vi "FIFO.vi"() -> ()   [LabVIEW 2019]
uses:
  <vilib>/rvi/Emulation/niFpgaGetClockAttributes.vi
  <vilib>/rvi/Emulation/niFpgaSctlEmulationGetInTimedLoop.vi
  <vilib>/rvi/Emulation/niFpgaEmulationReportErrorSimple.vi
  <vilib>/rvi/eio/common/nirviEmuTemplateMethod_errors.vi
  <vilib>/rvi/DataTransferAndStorage/Container/Common/niFpgaContainerExecOnDevCompGetState.vi
  <vilib>/rvi/Emulation/niFpgaEmulationIsFPGAContextNoSignature.vi
  <vilib>/rvi/errors/niFpgaSetErrorForExecOnDevCompSimple.vi
  <vilib>/rvi/eio/common/nirviEmuReportErrorAndStop.vi
  <vilib>/rvi/DataTransferAndStorage/Container/Common/niFpgaContainerGetUniqueNameForEmu.vi
  <vilib>/rvi/FIFO/Fifo_Resource/nirvififoEmulationSetSize.vi
  <vilib>/rvi/FIFO/Fifo_Resource/nirviFifoEmulationQueueMgr.vi
  <instcachedir>/0/nirviFifoEmulationQueueMgr_E5CAEC123FF24DC58D834DCA3CDAA9B5.lvgen/nirviFifoEmulationQueueMgr_E5CAEC123FF24DC58D834DCA3CDAA9B5_002.vi
  <vilib>/rvi/FIFO/Fifo_Resource/nirvififoEmulationDetermineInputValidOut.vi
  <vilib>/rvi/FIFO/Fifo_Resource/nirvififoEmulationCreateLock.vi
  <vilib>/rvi/Emulation/niFpgaProcessEmulError.vi
  <vilib>/rvi/FIFO/Fifo_Resource/nirvififoEmulationObtainLock.vi
  <vilib>/rvi/FIFO/Fifo_Resource/nirvififoEmulationReleaseLock.vi
  <vilib>/rvi/occurrence/nirviWaitOnOccurrenceBase.vi
  <vilib>/rvi/errors/nirviReportUnexpectedCaseInternalError.vi
  <vilib>/rvi/errors/nirviReportUnexpectedCaseInternalError (U32).vi
  <vilib>/Utility/error.llb/Clear Errors.vi
  <vilib>/rvi/interface/RandomDataEmulation/niFpgaRandomDataHandleErrors.vi
  <instcachedir>/0/nirviFifoEmulationQueueMgr_E5CAEC123FF24DC58D834DCA3CDAA9B5.lvgen/nirviFifoEmulationQueueMgr_E5CAEC123FF24DC58D834DCA3CDAA9B5_000.vi
  <instcachedir>/0/nirviFifoEmulationQueueMgr_E5CAEC123FF24DC58D834DCA3CDAA9B5.lvgen/nirviFifoEmulationQueueMgr_E5CAEC123FF24DC58D834DCA3CDAA9B5_001.vi
  <vilib>/rvi/Emulation/niFpgaCriticalErrorInLSC.vi
  <vilib>/eio/EIONode/EIONode.xnode
  <vilib>/rvi/DataTransferAndStorage/Container/XNode/niFpgaContainer.xnode
  <vilib>/rvi/FIFO/Fifo_Resource/niFpgaFifoEmulationRefIn.vi
panel:
  out "Laser":i16
  in  "stop":bool
  out "volt":i16
  out "Count":u32 caption="Tick Count(uSec)"
  out "Load":u16
  in  "Count(uSec)":u32
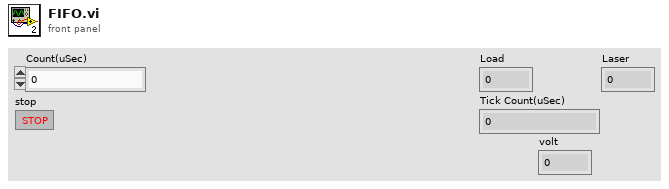
[diagram p1: front panel]
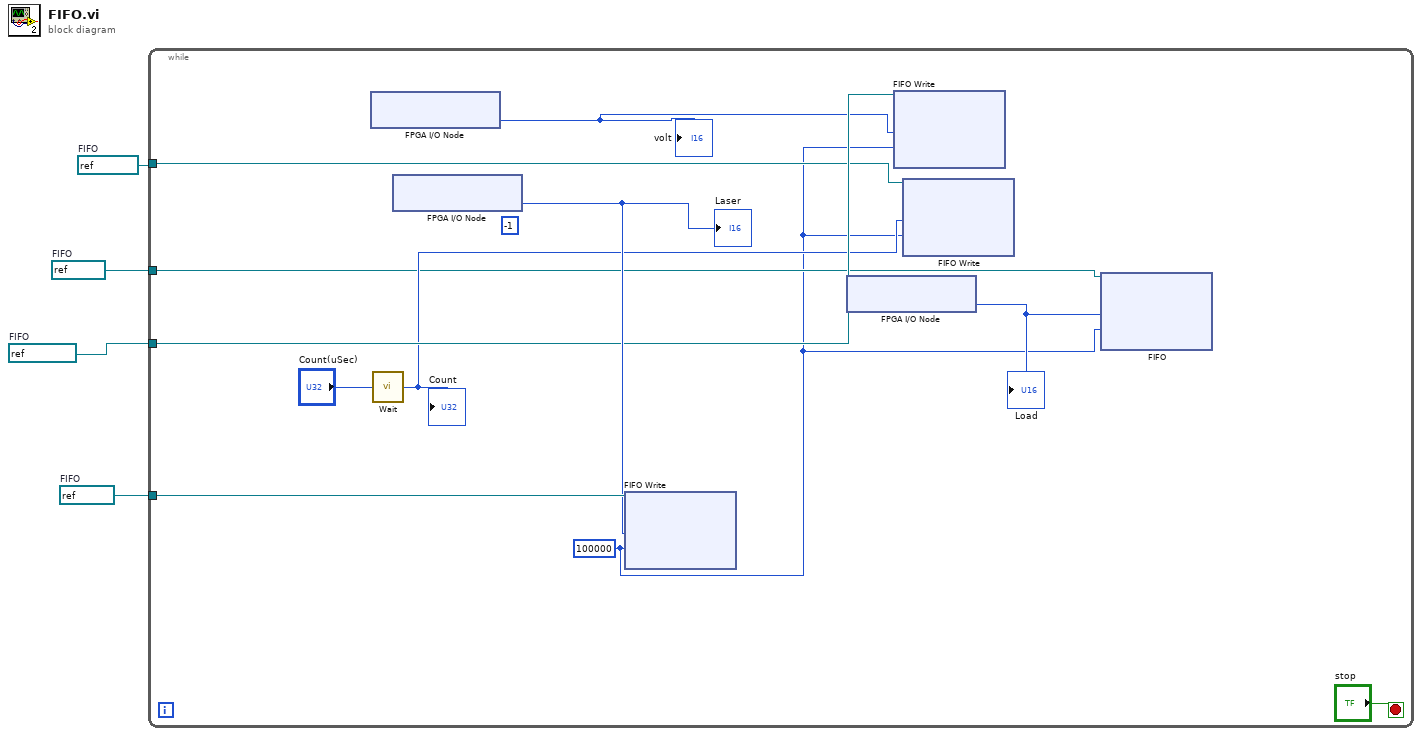
[diagram p0: block diagram]
diagram:
  w1 = refnum<k21> "Load"  # FIFO
  w2 = refnum<k21> "Count"  # FIFO
  w3 = refnum<k21> "Voltage"  # FIFO
  w4 = refnum<k21> "Laser"  # FIFO
  n1 = while {
    tunnel: w4 -> [w13]
    tunnel: w3 -> [w11]
    tunnel: w2 -> [w9]
    tunnel: w1 -> [w7]
    stop <- "stop" stop-if-true
    w5 = 100000 ("Timeout")
    (unwired) -1
    n2 = xnode "FPGA I/O Node"() -> ("ConnectorC/AI0"=w10:i16)  [unwired: 1 in, 1 out]
    "volt" <- w10
    n3 = call "Wait"("Count(uSec)"="Count(uSec)") -> ("Tick Count(uSec)"=w8:u32)
    "Count" <- w8
    n4 = xnode "FPGA I/O Node"() -> ("ConnectorC/AI1"=w12:i16)  [unwired: 1 in, 1 out]
    "Laser" <- w12
    n5 = xnode ("FIFO Write")("Element"=w12, "Timeout"=w5, "FIFO In"=w13) -> ()  [unwired: 2 out]
    n6 = xnode "FPGA I/O Node"() -> ("ConnectorA/AI1"=w6:u16)  [unwired: 1 in, 1 out]
    "Load" <- w6
    n7 = xnode ("FIFO Write")("Element"=w10, "Timeout"=w5, "FIFO In"=w11) -> ()  [unwired: 2 out]
    n8 = xnode ("FIFO Write")("Element"=w8, "Timeout"=w5, "FIFO In"=w9) -> ()  [unwired: 2 out]
    n9 = xnode "FIFO"("Element"=w6, "Timeout"=w5, "FIFO In"=w7) -> ()  [unwired: 2 out]
  }
